vi "Crop Video Utility.vi"() -> ()   [LabVIEW 2017]
uses:
  LabVIEW/Controls/Time Crop Method.ctl
  LabVIEW/Controls/Annotation Type.ctl
  LabVIEW/Controls/Crop Video State.ctl
  LabVIEW/Controls/Frame Grabber Data.ctl
  <vilib>/userdefined/High Color/IMAQdx.ctl
  <vilib>/vision/Image Controls.llb/IMAQ Image.ctl
  <vilib>/vision/Avi.llb/IMAQ AVI2 Refnum.ctl
  LabVIEW/Controls/Rigid Body Info.ctl
  LabVIEW/Controls/Position.ctl
  LabVIEW/Controls/Orientation.ctl
  LabVIEW/Controls/Refnums.ctl
  LabVIEW/Controls/Dimensions.ctl
  LabVIEW/Controls/Room Dimensions.ctl
panel:
  in  "Continuous Playback":bool
  out "Number of Camera Frames":u32
  out "Camera Frame":u32
  in  "Clip Width":i32=1 caption="+/-" min=1
  in  "Annotation Type":T1 caption="Type"
  in  "Annotate":bool
  in  "Annotation":string
  out "Time elapsed (s)":dbl format="%_4g"
  in  "Step Size":i32=100
  in  "Skip Backward":bool
  in  "Skip Forward":bool
  in  "Invert Playback?":bool
  out "Cancel Save":bool
  in  "Time Crop\nMethod":T2
  in  "Save":bool
  in  "Help Crop":bool
  in  "Load":bool
  in  "Stop":bool
  out "Ultrasound Frame":T3(plugin-control)
  in  "Play":bool
  out "Video path":path
  out "Number of Playback Frames":i32
  in  "Playback Rate":dbl(knob)=10.173051878092375 min=1.0 max=100.0 scale=1.0..100.0
  in  "Frame Slider":cluster{i32, i32, i32}(slide)={0, 100, 0} scale=0.0..17201.0
  out "Saving":bool
  in  "Codec":u16(ring)=3 items=["Cinepak Codec by Radius", "Intel IYUV codec", "Microsoft Video 1", "FF Video Codec 1 (FFV1) (NI Vision)", "Motion JPEG (NI Vision)", "Y800 Uncompressed Grey Scale (NI Vision)", "YUV 4:2:0 Planar (NI Vision)"]
  in  "Set Crop Area":bool
  in  "Clear Crop Area":bool
  # "of"
  # "of"
  # "Min"
  # "Max"
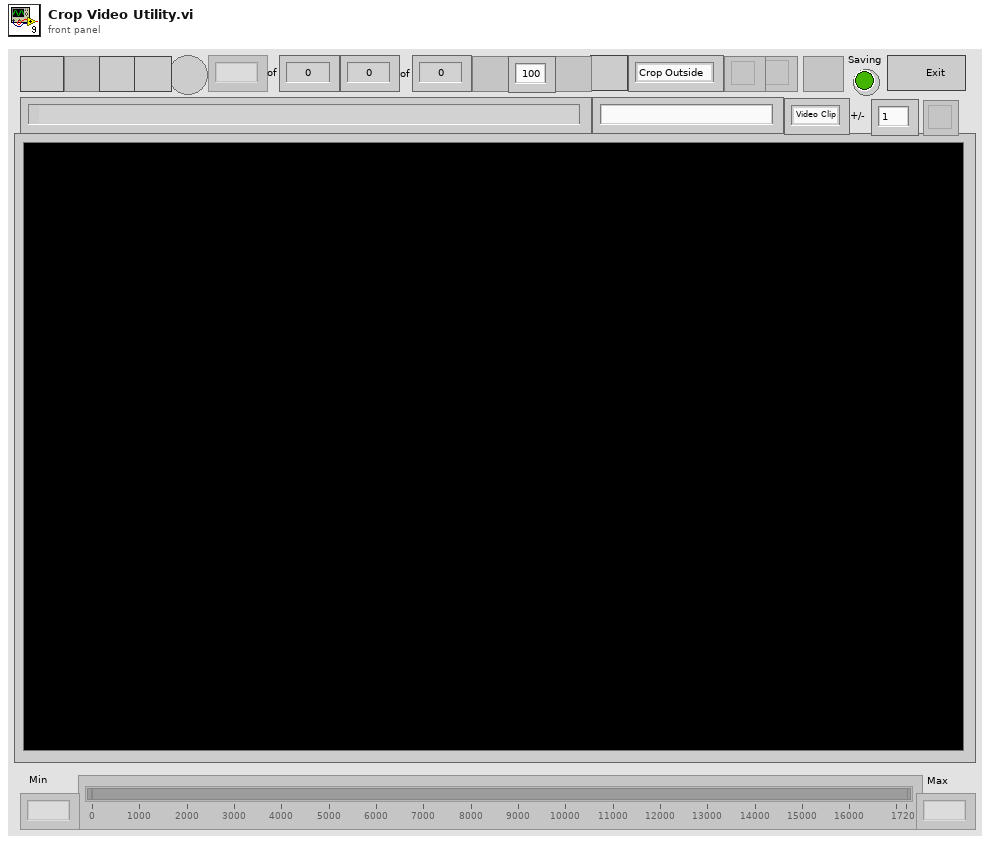
[diagram p1: front panel]
types:
  T1 = typedef "Annotation Type.ctl" = enum16{"Video Clip", "Image"}
  T2 = typedef "Time Crop Method.ctl" = enum16{"Crop Outside", "Crop Inside"}
  T3 = typedef "IMAQ Image.ctl" = refnum<image>
  T4 = typedef "Frame Grabber Data.ctl" = cluster{"Camera Session":T5, "Frame":T3, "AVI Refnum":T6, "Codecs":string[], "Frame number":u32, "Tracking File Refnum":refnum<file>, "Tick Count":u32, "Probe Object":refnum<vi>, "Playback Probe Data":dbl[][], "Rigid Body":T7, "Total no frames playback":i32, "Video FPS":dbl, "Camera connected?":bool, "Scene":refnum<vi>, "Cropped Frame":T3, "Tracker FPS":dbl, "Crop ROI":i32[], "Presentation Values":string[], "Elapsed time (ms)":u32, "Camera frames playback":u32, "Refnums":T10, "Dimensions":T11, "Playback Data As Strings":string[][], "Cropped Tracking File Refnum":refnum<file>, "Cropped AVI Refnum":T6, "Header":string[], "Total euclidian distance":dbl, "Annotation File Path":path, "Playback File Path":path, "Size per frame":dbl}
  T5 = typedef "IMAQdx.ctl" = refnum<k21>
  T6 = typedef "IMAQ AVI2 Refnum.ctl" = refnum<k20>
  T7 = typedef "Rigid Body Info.ctl" = cluster{"Position":T8, "Orientation":T9, "Quaternion":cluster{"qx":sgl, "qy":sgl, "qz":sgl, "qw":sgl}, "Tracked?":bool}
  T8 = typedef "Position.ctl" = cluster{"x (mm)":sgl, "y (mm)":sgl, "z (mm)":sgl}
  T9 = typedef "Orientation.ctl" = cluster{"Pitch (rad)":sgl, "Yaw (rad)":sgl, "Roll (rad)":sgl}
  T10 = typedef "Refnums.ctl" = cluster{"Live Refnum":refnum<vi>, "Record Refnum":refnum<vi>, "Playback Refnum":refnum<vi>, "Frame Slider Refnum":refnum<vi>, "Pause Refnum":refnum<vi>, "Home Refnum":refnum<vi>, "Crop Refnum":refnum<vi>, "Clear Crop Refnum":refnum<vi>, "stop refnum":refnum<vi>, "Playback Rate Refnum":refnum<vi>, "Presentation Refnum":refnum<vi>, "Crop Time Frame Slider Refnum":refnum<vi>, "Cancel Save Refnum":refnum<vi>, "Reverse Playback Refnum":refnum<vi>, "Recording Settings Refnum":refnum<vi>, "Camera Frame Refnum":refnum<vi>, "Continuous Playback Refnum":refnum<vi>}
  T11 = typedef "Dimensions.ctl" = cluster{"Probe Dimensions":cluster{"Probe Width":sgl, "Probe Depth":sgl, "Probe Height":sgl}, "Room Dimensions":T12}
  T12 = typedef "Room Dimensions.ctl" = cluster{"Room Width":dbl, "Room Depth":dbl, "Room Height":dbl}
  T13 = typedef "Crop Video State.ctl" = enum16{"Init", "Wait", "Load", "Playback Frame", "Save", "Close", "Set Crop Area", "Reset Crop Area", "Crop Inside", "Crop Outside", "Annotate Frame", "Annotate Clip", "Error Handling", "Shutdown"}
  T14 = typedef "Semaphore RefNum" = refnum<k1>
  T15 = enum8{"Enabled", "Disabled", "Disabled and Grayed Out"}
  T16 = typedef "Image Type" = u32
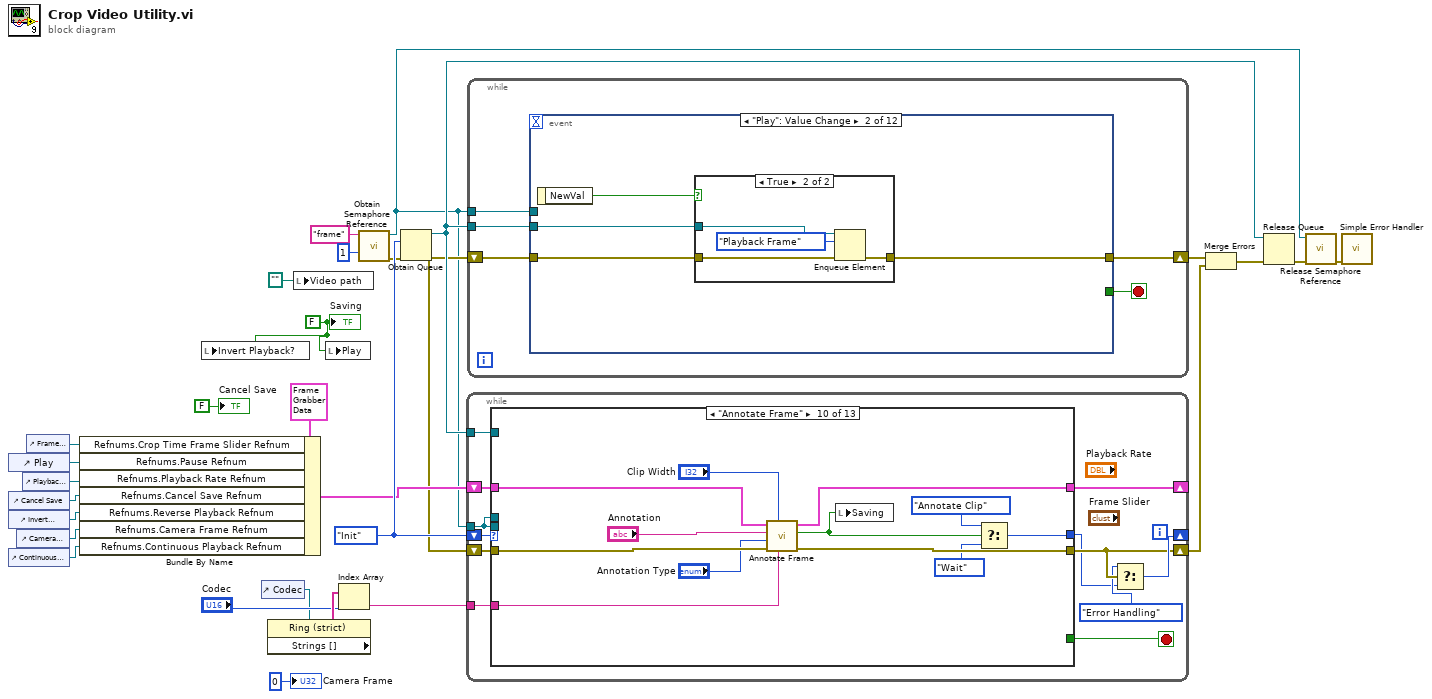
[diagram p0: block diagram]
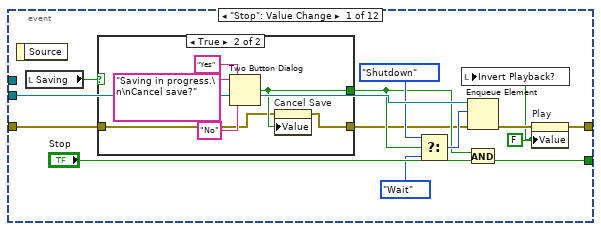
[diagram p2: hidden frame]
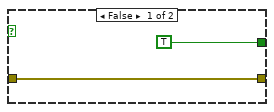
[diagram p3: hidden frame]
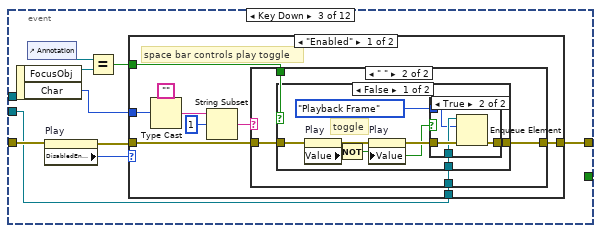
[diagram p5: hidden frame]
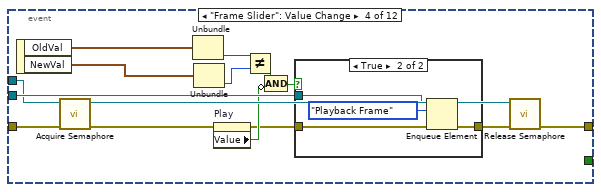
[diagram p10: hidden frame]
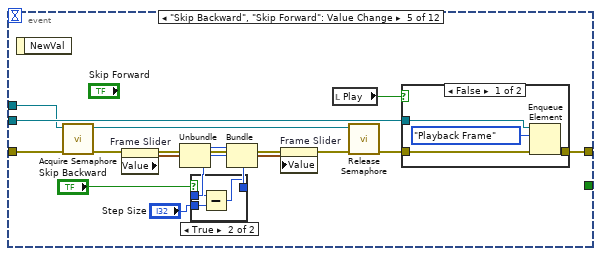
[diagram p12: hidden frame]
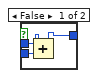
[diagram p14: hidden frame]
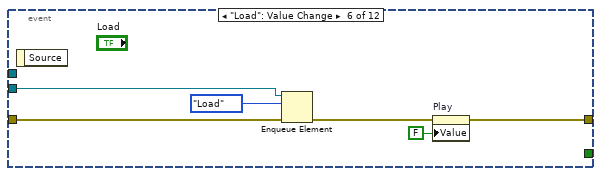
[diagram p15: hidden frame]
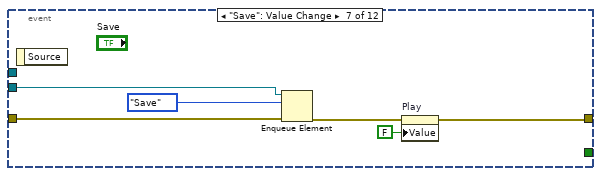
[diagram p16: hidden frame]
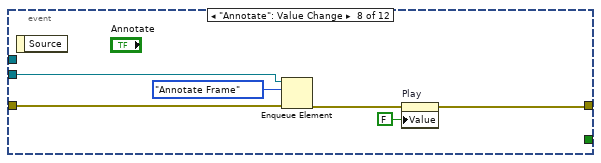
[diagram p17: hidden frame]
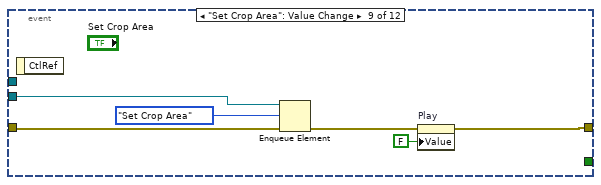
[diagram p18: hidden frame]
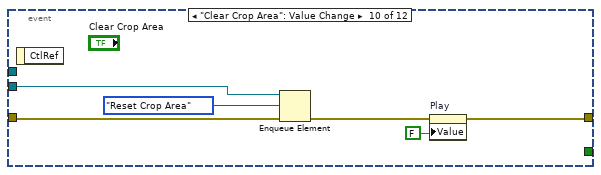
[diagram p19: hidden frame]
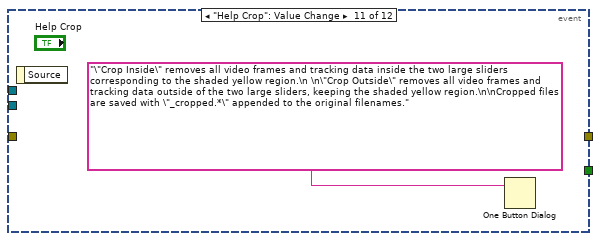
[diagram p20: hidden frame]
diagram:
  w29 = Crop_Video_State."Init" ("State")
  w11 = FALSE ("Saving")
  n1 = control-ref of="Play"() -> (w24:refnum<vi>)
  n2 = control-ref of="Cancel Save"() -> (w12:refnum<vi>)
  n3 = control-ref of="Invert Playback?"() -> (w10:refnum<vi>)
  n4 = control-ref of="Continuous Playback"() -> (w1:refnum<vi>)
  n5 = control-ref of="Camera Frame"() -> (w3:refnum<vi>)
  n6 = control-ref of="Playback Rate"() -> (w23:refnum<vi>)
  n7 = control-ref of="Frame Slider"() -> (w18:refnum<vi>)
  n8 = Bundle By Name(cluster=T4 {"Camera Session"="", "Frame"=refnum, "AVI Refnum"=refnum, "Codecs"=[], "Frame number"=0, "Tracking File Refnum"=refnum, "Tick Count"=0, "Probe Object"=refnum, "Playback Probe Data"=[], "Rigid Body"={"Position"={"x (mm)"=0.0, "y (mm)"=0.0, "z (mm)"=0.0}, "Orientation"={"Pitch (rad)"=0.0, "Yaw (rad)"=0.0, "Roll (rad)"=0.0}, "Quaternion"={"qx"=0.0, "qy"=0.0, "qz"=0.0, "qw"=0.0}, "Tracked?"=FALSE}, "Total no frames playback"=0, "Video FPS"=0.0, "Camera connected?"=FALSE, "Scene"=refnum, "Cropped Frame"=refnum, "Tracker FPS"=0.0, "Crop ROI"=[], "Presentation Values"=[], "Elapsed time (ms)"=0, "Camera frames playback"=0, "Refnums"={"Live Refnum"=refnum, "Record Refnum"=refnum, "Playback Refnum"=refnum, "Frame Slider Refnum"=refnum, "Pause Refnum"=refnum, "Home Refnum"=refnum, "Crop Refnum"=refnum, "Clear Crop Refnum"=refnum, "stop refnum"=refnum, "Playback Rate Refnum"=refnum, "Presentation Refnum"=refnum, "Crop Time Frame Slider Refnum"=refnum, "Cancel Save Refnum"=refnum, "Reverse Playback Refnum"=refnum, "Recording Settings Refnum"=refnum, "Camera Frame Refnum"=refnum, "Continuous Playback Refnum"=refnum}, "Dimensions"={"Probe Dimensions"={"Probe Width"=0.0, "Probe Depth"=1.0, "Probe Height"=0.0}, "Room Dimensions"={"Room Width"=0.0, "Room Depth"=0.0, "Room Height"=0.0}}, "Playback Data As Strings"=[], "Cropped Tracking File Refnum"=refnum, "Cropped AVI Refnum"=refnum, "Header"=[], "Total euclidian distance"=0.0, "Annotation File Path"=path "", "Playback File Path"=path "", "Size per frame"=0.0} ("Frame Grabber Data 2"), "Refnums.Crop Time Frame Slider Refnum"=w18, "Refnums.Pause Refnum"=w24, "Refnums.Playback Rate Refnum"=w23, "Refnums.Cancel Save Refnum"=w12, "Refnums.Reverse Playback Refnum"=w10, "Refnums.Camera Frame Refnum"=w3, "Refnums.Continuous Playback Refnum"=w1) -> (w21:T4)
  n9 = local write "Invert Playback?"(w11) -> ()
  n10 = control-ref of="Codec"() -> (w14:refnum<vi>)
  n11 = property class="Ring (strict)"(reference=w14) -> ("Strings []"=w17:string[])  [unwired: 1 in, 2 out]
  n12 = local write "Video path"(path "") -> ()
  n13 = local write "Play"(w11) -> ()
  n14 = Index Array(array=w17, index="Codec") -> (element=w16:string)
  n15 = call <vilib>:"Obtain Semaphore Reference.vi"("size (1)"=1, "name (unnamed)"="frame") -> ("error out"=w6:errorcluster, "semaphore"=w4:T14)  [unwired: 3 in, 1 out]
  n16 = Obtain Queue(element data type=w29, error in (no error)=w6) -> (queue out=w25:refnum<queue>, error out=w20:errorcluster)  [unwired: 3 in, 1 out]
  n17 = while {
    shift-right: [w36] -> _
    shift-left: w21 -> [w37]
    tunnel: w25 -> [w39]
    shift-right: [w34] -> w27
    shift-left: w20 -> [w38]
    shift-right: [w35] -> _
    shift-left: w29 -> [w41]
    tunnel: w16 -> [w32]
    tunnel: w4 -> [w30]
    stop <- w40 stop-if-true
    n18 = case shown="\"Annotate Frame\"" w41 {
      selector: w41 -> [_ _ _ _ _ _ _ _ _ _ w272 _ w311]
      tunnel: [_ _ _ _ _ _ _ _ _ _ _ _ w304] -> w40
      tunnel: w39 -> [_ w69 _ _ _ _ _ _ _ _ _ _ _]
      tunnel: w38 -> [w54 w68 w83 w118 w126 w135 w173 w193 w226 w255 w276 w293 w308]
      tunnel: [w55 w67 w76 w112 w121 w131 w167 w207 w233 w254 w279 w291 w310] -> w34
      tunnel: [Crop_Video_State."Wait" ("State") w66 w75 Crop_Video_State."Wait" ("State") Crop_Video_State."Wait" ("State") w140 w166 Crop_Video_State."Close" ("State") Crop_Video_State."Close" ("State") w248 Crop_Video_State."Wait" ("State") Crop_Video_State."Close" ("State") Crop_Video_State."Wait" ("State")] -> w31
      tunnel: w37 -> [w62 w65 w78 w117 w124 w138 w174 w195 w232 w252 w273 w288 w312]
      tunnel: [w59 w65 w80 w116 w125 w137 w171 w209 w235 w251 w267 w288 w303] -> w36
      tunnel: w32 -> [_ _ _ _ _ _ w172 _ _ w244 _ _ _]
      tunnel: w30 -> [_ _ _ _ _ _ _ _ _ _ _ _ _]
      tunnel: w30 -> [_ _ _ _ _ w132 _ _ _ _ _ _ _]
      frame "Init" {
        w48 = T15."Disabled and Grayed Out" ("Disabled")
        w53 = u32 100 ("Frame")
        w52 = u32 0 ("Min")
        w42 = T16 4 items=["Grayscale (U8)", "Grayscale (I16)", "Grayscale (SGL)", "Complex (CSG)", "RGB (U32)", "HSL (U32)", "RGB (U64)", "Grayscale (U16)"] ("Image Type")
        n19 = property on="Play" class="Bool (strict)"(error in=w54, "DisabledEnum"=w48) -> (error out=w51:errorcluster)  [unwired: 1 in, 1 out]
        n20 = property on="Set Crop Area" class="Bool"(error in=w51, "DisabledEnum"=w48) -> (error out=w50:errorcluster)  [unwired: 1 in, 1 out]
        n21 = property on="Clear Crop Area" class="Bool"(error in=w50, "DisabledEnum"=w48) -> (error out=w49:errorcluster)  [unwired: 1 in, 1 out]
        n22 = property on="Save" class="Bool"(error in=w49, "DisabledEnum"=w48) -> (error out=w47:errorcluster)  [unwired: 1 in, 1 out]
        n23 = property on="Frame Slider" class="Slide (strict)"(error in=w47, "DisabledEnum"=w48) -> (error out=w46:errorcluster)  [unwired: 1 in, 1 out]
        n24 = call "IMAQ Create"("Image Name"="cropped frame", "Image Type"=w42, "error in (no error)"=w46) -> ("New Image"=w43:T3, "error out"=w45:errorcluster)  [unwired: 2 in]
        n25 = Bundle(cluster=cluster{"Min":u32, "Max":u32, "Frame":u32} {"Min"=24, "Max"=167, "Frame"=33} ("Frame Slider"), "Min"=w52, "Max"=w53, "Frame"=w52) -> (w58:cluster{"Min":u32, "Max":u32, "Frame":u32})
        n26 = call "IMAQ Create"("Image Name"="frame", "Image Type"=w42, "error in (no error)"=w45) -> ("New Image"=w61:T3, "error out"=w56:errorcluster)  [unwired: 2 in]
        n27 = Bundle By Name(cluster=w62, "Cropped Frame"=w43, "Frame"=w61) -> (w59:T4)
        n28 = property on="Frame Slider" class="Slide (strict)"(error in=w56, "Value"=w58, "Scale.Minimum"=w52, "Scale.Maximum"=w53) -> (error out=w55:errorcluster)  [unwired: 1 in, 1 out]
      }
      frame "Wait", Default {
        n29 = local write "Play"(FALSE) -> ()
        n30 = Dequeue Element(queue=w69, error in (no error)=w68) -> (element=w66:T13, error out=w67:errorcluster)  [unwired: 1 in, 2 out]
      }
      frame "Load" {
        n31 = call "Open Playback Files Cropping.vi"("error in (no error)"=w83, "Frame Grabber Data In"=w78) -> ("error out"=w81:errorcluster, "Playback Video"=w82:path, "both exist and open?"=w77:bool, "Frame Grabber Data Out"=w79:T4, "Number of Playback Frames"=w74:i32, "Number of Camera Frames"=w71:u32)  [unwired: 4 in]
        n32 = Decrement(x=w71) -> (x-1=→"Number of Camera Frames":u32)
        n33 = Decrement(x=w74) -> (x-1=→"Number of Playback Frames":i32)
        n34 = case shown="True" w77 {
          tunnel: w82 -> [w87 _]
          tunnel: w81 -> [w90 w103]
          tunnel: [w96 w109] -> w80
          tunnel: w79 -> [w96 w109]
          tunnel: w78 -> [_ _]
          tunnel: [w85 w99] -> w76
          tunnel: [Crop_Video_State."Playback Frame" ("State") Crop_Video_State."Wait" ("State")] -> w75
          tunnel: [w87 _] -> w73
          frame True {
            w84 = T15."Enabled" ("Disabled")
            n35 = property on="Skip Backward" class="Bool"(error in=w90, "DisabledEnum"=w84) -> (error out=w89:errorcluster)  [unwired: 1 in, 1 out]
            n36 = property on="Skip Forward" class="Bool"(error in=w89, "DisabledEnum"=w84) -> (error out=w88:errorcluster)  [unwired: 1 in, 1 out]
            n37 = property on="Play" class="Bool (strict)"(error in=w88, "DisabledEnum"=w84) -> (error out=w93:errorcluster)  [unwired: 1 in, 1 out]
            n38 = property on="Set Crop Area" class="Bool"(error in=w93, "DisabledEnum"=w84) -> (error out=w92:errorcluster)  [unwired: 1 in, 1 out]
            n39 = property on="Save" class="Bool"(error in=w92, "DisabledEnum"=w84) -> (error out=w91:errorcluster)  [unwired: 1 in, 1 out]
            n40 = local write "Play"(TRUE ("Play")) -> ()
            n41 = property on="Frame Slider" class="Slide (strict)"(error in=w91, "DisabledEnum"=w84) -> (error out=w86:errorcluster)  [unwired: 1 in, 1 out]
            n42 = property on="Annotate" class="Bool"(error in=w86, "DisabledEnum"=w84) -> (error out=w85:errorcluster)  [unwired: 1 in, 1 out]
          }
          frame False {
            w97 = T15."Disabled and Grayed Out" ("Disabled")
            n43 = property on="Skip Backward" class="Bool"(error in=w103, "DisabledEnum"=w97) -> (error out=w102:errorcluster)  [unwired: 1 in, 1 out]
            n44 = property on="Skip Forward" class="Bool"(error in=w102, "DisabledEnum"=w97) -> (error out=w101:errorcluster)  [unwired: 1 in, 1 out]
            n45 = property on="Play" class="Bool (strict)"(error in=w101, "DisabledEnum"=w97) -> (error out=w106:errorcluster)  [unwired: 1 in, 1 out]
            n46 = property on="Set Crop Area" class="Bool"(error in=w106, "DisabledEnum"=w97) -> (error out=w105:errorcluster)  [unwired: 1 in, 1 out]
            n47 = property on="Save" class="Bool"(error in=w105, "DisabledEnum"=w97) -> (error out=w104:errorcluster)  [unwired: 1 in, 1 out]
            n48 = One Button Dialog(message="Could not open files for playback.") -> ()  [unwired: 1 in, 1 out]
            n49 = local write "Play"(TRUE ("Play")) -> ()
            n50 = property on="Frame Slider" class="Slide (strict)"(error in=w104, "DisabledEnum"=w97) -> (error out=w98:errorcluster)  [unwired: 1 in, 1 out]
            n51 = property on="Annotate" class="Bool"(error in=w98, "DisabledEnum"=w97) -> (error out=w99:errorcluster)  [unwired: 1 in, 1 out]
          }
        }
        "Video path" <- w73
      }
      frame "Set Crop Area" {
        n52 = call "Set Crop ROI.vi"("error in (no error)"=w118, "Frame Grabber Data in"=w117) -> ("error out"=w110:errorcluster, "Image Out"=w115:T3, "Frame Grabber Data out"=w116:T4, "Zero crop size?"=w111:bool)  [unwired: 5 in, 1 out]
        n53 = local write "Ultrasound Frame"(w115) -> ()
        n54 = case shown="True" w111 {
          frame False {
          }
          frame True {
            n55 = One Button Dialog(message="Warning: invalid crop area.") -> ()  [unwired: 1 in, 1 out]
          }
        }
        n56 = property on="Clear Crop Area" class="Bool"(error in=w110, "DisabledEnum"=T15."Enabled" ("Disabled")) -> (error out=w112:errorcluster)  [unwired: 1 in, 1 out]
      }
      frame "Reset Crop Area" {
        n57 = call "Clear Crop ROI.vi"("error in (no error)"=w126, "Frame Grabber Data in"=w124) -> ("error out"=w121:errorcluster, "Image Out"=w123:T3, "Frame Grabber Data out"=w125:T4)  [unwired: 6 in, 1 out]
        n58 = local write "Ultrasound Frame"(w123) -> ()
        n59 = property on="Clear Crop Area" class="Bool"(error in=w121, "DisabledEnum"=T15."Disabled and Grayed Out" ("Disabled")) -> ()  [unwired: 1 in, 2 out]
      }
      frame "Playback Frame" {
        n60 = call "Playback Frame Cropping.vi"("error in (no error)"=w135, "Frame Grabber Data in"=w138) -> ("error out"=w133:errorcluster, "Continue playback?"=w130:bool, "Image"=→"Ultrasound Frame":T3, "Frame Grabber Data out"=w137:T4, "Time elapsed (s)"=→"Time elapsed (s)":dbl)  [unwired: 4 in, 1 out]
        n61 = case shown="True" w130 {
          selector: w130 -> [w143 w145]
          tunnel: [w144 w147] -> w131
          tunnel: "Invert Playback?" -> [_ w152]
          tunnel: w133 -> [w144 w151]
          tunnel: w132 -> [_ w150]
          tunnel: [w143 w145] -> w129
          frame False {
          }
          frame True {
            n62 = call <vilib>:"Acquire Semaphore.vi"("error in (no error)"=w151, "semaphore"=w150) -> ("error out"=w149:errorcluster, "semaphore out"=w146:T14)  [unwired: 3 in, 1 out]
            n63 = property on="Frame Slider" class="Slide (strict)"(error in=w149) -> (error out=w155:errorcluster, "Value"=w158:cluster{i32, i32, i32})  [unwired: 1 in, 1 out]
            n64 = Unbundle(w158) -> (w157:i32, w156:i32, w154:i32)
            n65 = case shown="True" w152 {
              tunnel: w154 -> [w161 w162]
              tunnel: [w160 w163] -> w153
              frame False {
                n66 = Increment(x=w161) -> (x+1=w160:i32)
              }
              frame True {
                n67 = Decrement(x=w162) -> (x-1=w163:i32)
              }
            }
            n68 = Bundle(w157, w156, w153) -> (w159:cluster{i32, i32, i32})  [unwired: 1 in]
            n69 = property on="Frame Slider" class="Slide (strict)"(error in=w155, "Value"=w159) -> (error out=w148:errorcluster)  [unwired: 1 in, 1 out]
            n70 = call <vilib>:"Release Semaphore.vi"("error in (no error)"=w148, "semaphore"=w146) -> ("error out"=w147:errorcluster)  [unwired: 4 in, 1 out]
          }
        }
        n71 = And(x="Play", y=w129) -> (x .and. y?=w128:bool)
        n72 = Select(t=Crop_Video_State."Playback Frame" ("State"), s=w128, f=Crop_Video_State."Wait" ("State")) -> (s? t:f=w140:T13)
      }
      frame "Save" {
        n73 = call "Configure Crop.vi"("Codec"=w172, "error in (no error)"=w173, "Time Crop Method"="Time Crop\nMethod", "Frame Grabber Data In"=w174) -> ("error out"=w169:errorcluster, "Valid crop region?"=w170:bool, "Saving?"=w164:bool, "Frame Grabber Data Out"=w171:T4)  [unwired: 4 in]
        n74 = local write "Saving"(w164) -> ()
        n75 = And(x=w164, y=w170) -> (x .and. y?=w165:bool)
        n76 = case shown="True" w165 {
          tunnel: w169 -> [w175 w187]
          tunnel: "Time Crop\nMethod" -> [_ w189]
          tunnel: [Crop_Video_State."Wait" ("State") w188] -> w166
          tunnel: [w175 w179] -> w167
          frame False {
            n77 = One Button Dialog(message="Invalid time crop region/save cancelled by user.") -> ()  [unwired: 1 in, 1 out]
          }
          frame True {
            w178 = T15."Disabled and Grayed Out" ("Disabled")
            n78 = property on="Set Crop Area" class="Bool"(error in=w187, "DisabledEnum"=w178) -> (error out=w186:errorcluster)  [unwired: 1 in, 1 out]
            n79 = property on="Save" class="Bool"(error in=w186, "DisabledEnum"=w178) -> (error out=w185:errorcluster)  [unwired: 1 in, 1 out]
            n80 = property on="Load" class="Bool"(error in=w185, "DisabledEnum"=w178) -> (error out=w184:errorcluster)  [unwired: 1 in, 1 out]
            n81 = property on="Frame Slider" class="Slide (strict)"(error in=w184, "DisabledEnum"=w178) -> (error out=w183:errorcluster)  [unwired: 1 in, 1 out]
            n82 = property on="Clear Crop Area" class="Bool"(error in=w183, "DisabledEnum"=w178) -> (error out=w181:errorcluster)  [unwired: 1 in, 1 out]
            n83 = property on="Load" class="Bool"(error in=w181, "DisabledEnum"=w178) -> (error out=w182:errorcluster)  [unwired: 1 in, 1 out]
            n84 = case shown="\"Crop Outside\", Default" w189 {
              tunnel: [Crop_Video_State."Crop Inside" ("t") Crop_Video_State."Crop Outside" ("t")] -> w188
              frame "Crop Inside" {
              }
              frame "Crop Outside", Default {
              }
            }
            n85 = property on="Play" class="Bool (strict)"(error in=w182, "DisabledEnum"=w178) -> (error out=w180:errorcluster)  [unwired: 1 in, 1 out]
            n86 = property on="Annotate" class="Bool"(error in=w180, "DisabledEnum"=w178) -> (error out=w179:errorcluster)  [unwired: 1 in, 1 out]
          }
        }
      }
      frame "Crop Inside" {
        w202 = u32 0 ("Starting frame number")
        n87 = property on="Frame Slider" class="Slide (strict)"(error in=w193) -> (error out=w192:errorcluster, "Value"=w194:cluster{i32, i32, i32})  [unwired: 1 in, 1 out]
        n88 = Bundle By Name(cluster=w195, "Frame number"=w202) -> (w196:T4)
        n89 = Unbundle By Name(w195) -> ("Total no frames playback"=w205:i32)
        n90 = Unbundle(w194) -> (w198:i32, w199:i32)  [unwired: 1 out]
        n91 = for {
          N: w198 -> [_]
          shift-right: [w220] -> w204
          shift-left: w192 -> [w221]
          shift-right: [w218] -> w201
          shift-left: w196 -> [w219]
          tunnel: w202 -> [w217]
          stop <- w216 stop-if-true
          # "First portion"
          n92 = call "Record Frame Crop.vi"("error in (no error)"=w221, "Starting frame number"=w217, "Frame Grabber Data In in"=w219) -> ("error out"=w220:errorcluster, "Cancel save?"=w216:bool, "Frame Grabber Data out"=w218:T4)  [unwired: 6 in]
        }
        n93 = Bundle By Name(cluster=w201, "Frame number"=w199) -> (w200:T4)
        n94 = Subtract(x=w199, y=w198) -> (x-y=w197:i32)
        n95 = Subtract(x=w205, y=w199) -> (x-y=w203:i32)
        n96 = for {
          N: w203 -> [_]
          shift-right: [w214] -> w208
          shift-left: w204 -> [w215]
          shift-right: [w212] -> w209
          shift-left: w200 -> [w213]
          tunnel: w197 -> [w211]
          stop <- w210 stop-if-true
          # "Second portion"
          n97 = call "Record Frame Crop.vi"("error in (no error)"=w215, "Starting frame number"=w211, "Frame Grabber Data In in"=w213) -> ("error out"=w214:errorcluster, "Cancel save?"=w210:bool, "Frame Grabber Data out"=w212:T4)  [unwired: 6 in]
        }
        n98 = flat-sequence {
          tunnel: w208 -> [w222]
          tunnel: [w222] -> w207
          frame #0 {
            n99 = local write "Saving"(FALSE) -> ()
          }
        }
      }
      frame "Crop Outside" {
        n100 = property on="Frame Slider" class="Slide (strict)"(error in=w226) -> (error out=w224:errorcluster, "Value"=w225:cluster{i32, i32, i32})  [unwired: 1 in, 1 out]
        n101 = Unbundle(w225) -> (w227:i32, w230:i32)  [unwired: 1 out]
        n102 = Bundle By Name(cluster=w232, "Frame number"=w227) -> (w228:T4)
        n103 = Subtract(x=w230, y=w227) -> (x-y=w229:i32)
        n104 = for {
          N: w229 -> [_]
          shift-right: [w240] -> w234
          shift-left: w224 -> [w241]
          tunnel: w227 -> [w239]
          shift-right: [w238] -> w235
          shift-left: w228 -> [w237]
          stop <- w236 stop-if-true
          # "Middle portion"
          n105 = call "Record Frame Crop.vi"("error in (no error)"=w241, "Starting frame number"=w239, "Frame Grabber Data In in"=w237) -> ("error out"=w240:errorcluster, "Cancel save?"=w236:bool, "Frame Grabber Data out"=w238:T4)  [unwired: 6 in]
        }
        n106 = flat-sequence {
          tunnel: w234 -> [w243]
          tunnel: [w243] -> w233
          frame #0 {
            n107 = local write "Saving"(FALSE) -> ()
          }
        }
      }
      frame "Annotate Frame" {
        n108 = call "Annotate Frame.vi"("Codec"=w244, "Clip width"="Clip Width", "error in (no error)"=w255, "Annotation Type"="Annotation Type", "Annotation"="Annotation", "Frame Grabber Data In in"=w252) -> ("error out"=w254:errorcluster, "saving?"=w250:bool, "Frame Grabber Data Out"=w251:T4)  [unwired: 3 in]
        n109 = local write "Saving"(w250) -> ()
        n110 = Select(t=Crop_Video_State."Annotate Clip" ("State"), s=w250, f=Crop_Video_State."Wait" ("State")) -> (s? t:f=w248:T13)
      }
      frame "Annotate Clip" {
        # "reset"
        n111 = local read "Clip Width"() -> (w266:i32)
        n112 = Unbundle By Name(w273) -> ("Tracker FPS"=w263:dbl, "Video FPS"=w262:dbl, "Frame number"=w259:u32)
        n113 = Multiply(x=w266, y=2) -> (x*y=w274:i32)
        n114 = To Double Precision Float(number=w259) -> (double precision float=w260:dbl)
        n115 = Divide(x=w263, y=w262) -> (x/y=w257:dbl)
        n116 = Quotient & Remainder(x=w260, y=w257) -> (floor(x/y)=w258:dbl)  [unwired: 1 out]
        n117 = Multiply(x=w257, y=w258) -> (x*y=w256:dbl)
        n118 = Multiply(x=w274, y=w257) -> (x*y=w264:dbl)
        n119 = Multiply(x=w266, y=w257) -> (x*y=w261:dbl)
        n120 = Subtract(x=w256, y=w261) -> (x-y=w265:dbl)
        n121 = Bundle By Name(cluster=w273, "Frame number"=w265) -> (w277:T4)
        n122 = for {
          N: w264 -> [_]
          shift-right: [w284] -> w271
          shift-left: w276 -> [w285]
          shift-right: [w283] -> w269
          shift-left: w277 -> [w282]
          stop <- w281 stop-if-true
          # "Middle portion"
          n123 = call "Record Frame Crop.vi"("error in (no error)"=w285, "Starting frame number"=u32 0, "Frame Grabber Data In in"=w282) -> ("error out"=w284:errorcluster, "Cancel save?"=w281:bool, "Frame Grabber Data out"=w283:T4)  [unwired: 6 in]
        }
        n124 = call "Close Files.vi"("error in (no error)"=w271, "State"=w272, "Frame Grabber Data in"=w269) -> ("error out"=w270:errorcluster, "Frame Grabber Data Out"=w268:T4)  [unwired: 5 in, 2 out]
        n125 = Bundle By Name(cluster=w268, "Frame number"=w259) -> (w267:T4)
        n126 = flat-sequence {
          tunnel: [w286] -> _
          tunnel: [w286] -> w279
          tunnel: w270 -> [w286]
          frame #0 {
            n127 = local write "Saving"(FALSE) -> ()
          }
        }
      }
      frame "Error Handling" {
        n128 = call <vilib>:"Simple Error Handler.vi"("error in (no error)"=w293) -> ("error out"=w292:errorcluster)  [unwired: 4 in, 4 out]
        n129 = local write "Play"(FALSE ("Play")) -> ()
        n130 = call <vilib>:"Clear Errors.vi"("error in (no error)"=w292) -> ("error out"=w291:errorcluster)  [unwired: 5 in, 1 out]
      }
      frame "Close", "Shutdown" {
        w295 = T15."Disabled and Grayed Out" ("Disabled")
        n131 = call "Close Files.vi"("error in (no error)"=w308, "State"=w311, "Frame Grabber Data in"=w312) -> ("error out"=w300:errorcluster, "Shutdown?"=w304:bool, "File Path Control"=w302:path, "Frame Grabber Data Out"=w303:T4)  [unwired: 5 in]
        n132 = property on="Skip Backward" class="Bool"(error in=w300, "DisabledEnum"=w295) -> (error out=w299:errorcluster)  [unwired: 1 in, 1 out]
        n133 = local write "Video path"(w302) -> ()
        n134 = local write "Camera Frame"(u32 0 ("Camera Frame")) -> ()
        n135 = property on="Skip Forward" class="Bool"(error in=w299, "DisabledEnum"=w295) -> (error out=w298:errorcluster)  [unwired: 1 in, 1 out]
        n136 = property on="Save" class="Bool"(error in=w298, "DisabledEnum"=w295) -> (error out=w307:errorcluster)  [unwired: 1 in, 1 out]
        n137 = property on="Clear Crop Area" class="Bool"(error in=w307, "DisabledEnum"=w295) -> (error out=w306:errorcluster)  [unwired: 1 in, 1 out]
        n138 = property on="Set Crop Area" class="Bool"(error in=w306, "DisabledEnum"=w295) -> (error out=w305:errorcluster)  [unwired: 1 in, 1 out]
        n139 = property on="Frame Slider" class="Slide (strict)"(error in=w305, "DisabledEnum"=w295) -> (error out=w301:errorcluster)  [unwired: 1 in, 1 out]
        n140 = property on="Play" class="Bool (strict)"(error in=w301, "DisabledEnum"=w295) -> (error out=w297:errorcluster)  [unwired: 1 in, 1 out]
        n141 = property on="Annotate" class="Bool"(error in=w297, "DisabledEnum"=w295) -> (error out=w296:errorcluster)  [unwired: 1 in, 1 out]
        n142 = property on="Load" class="Bool"(error in=w296, "DisabledEnum"=T15."Enabled" ("Disabled")) -> (error out=w310:errorcluster)  [unwired: 1 in, 1 out]
      }
    }
    n143 = Select(t=Crop_Video_State."Error Handling", s=w34, f=w31) -> (s? t:f=w35:T13)
  }
  n144 = while {
    tunnel: w25 -> [w317]
    shift-right: [w315] -> w28
    shift-left: w20 -> [w316]
    tunnel: w4 -> [w314]
    stop <- w318 stop-if-true
    n145 = event shown="[1] \"Play\": Value Change" {
      selector: _ -> [_ _ _ _ _ _ _ _ _ _ _ _]
      dyn-events: _ -> [_ _ _ _ _ _ _ _ _ _ _ _]
      timeout: _ -> [_ _ _ _ _ _ _ _ _ _ _ _]
      tunnel: [w323 _ _ _ _ _ _ _ _ _ _ _] -> w318
      tunnel: w317 -> [w330 w341 w352 w399 w424 w440 w446 w452 w459 w465 _ _]
      tunnel: w316 -> [w321 w343 w355 w398 w422 w441 w447 w453 w457 w463 _ w476]
      tunnel: [w329 w342 w356 w394 w411 w436 w443 w450 w454 w460 _ w475] -> w315
      tunnel: w314 -> [_ _ _ w397 w423 _ _ _ _ _ _ _]
      event "Stop": Value Change {
        w319 = FALSE ("Play")
        n146 = event-data() -> ()  [unwired: 1 in, 1 out]
        n147 = local read "Saving"() -> (w327:bool)
        n148 = case shown="True" w327 {
          tunnel: [TRUE ("T button?") w336] -> w322
          tunnel: w321 -> [w332 w335]
          tunnel: [w332 w334] -> w320
          frame False {
          }
          frame True {
            n149 = Two Button Dialog(message="Saving in progress.\n\nCancel save?", 1:"No" ("F button name (\"Cancel\")"), 2:"Yes" ("T button name (\"OK\")")) -> (T button?=w336:bool)
            n150 = property on="Cancel Save" class="Bool (strict)"(error in=w335, "Value"=w336) -> (error out=w334:errorcluster)  [unwired: 1 in, 1 out]
          }
        }
        n151 = Select(t=Crop_Video_State."Shutdown" ("element"), s=w322, f=Crop_Video_State."Wait") -> (s? t:f=w325:T13)
        n152 = local write "Invert Playback?"(w319) -> ()
        n153 = Enqueue Element(queue=w330, element=w325, error in (no error)=w320) -> (error out=w328:errorcluster)  [unwired: 1 in, 2 out]
        n154 = And(x=w322, y="Stop") -> (x .and. y?=w323:bool)
        n155 = property on="Play" class="Bool (strict)"(error in=w328, "Value"=w319) -> (error out=w329:errorcluster)  [unwired: 1 in, 1 out]
      }
      event "Play": Value Change {
        n156 = event-data() -> ("NewVal"=w340:bool)  [unwired: 1 in]
        n157 = case shown="True" w340 {
          tunnel: w343 -> [w344 w348]
          tunnel: [w344 w347] -> w342
          tunnel: w341 -> [_ w346]
          frame False {
          }
          frame True {
            n158 = Enqueue Element(queue=w346, element=Crop_Video_State."Playback Frame", error in (no error)=w348) -> (error out=w347:errorcluster)  [unwired: 1 in, 2 out]
          }
        }
      }
      event Key Down {
        n159 = event-data() -> ("FocusObj"=w351:refnum<vi>, "Char"=w357:i16)  [unwired: 1 in]
        n160 = control-ref of="Annotation"() -> (w350:refnum<vi>)
        n161 = property on="Play" class="Bool (strict)"(error in=w355) -> (error out=w354:errorcluster, "DisabledEnum"=w353:T15)  [unwired: 1 in, 1 out]
        n162 = Equal?(x=w350, y=w351) -> (x = y?=w349:bool)
        n163 = case shown="\"Enabled\"" w353 {
          tunnel: w357 -> [w364 _]
          tunnel: w354 -> [w361 w386]
          tunnel: [w360 w386] -> w356
          tunnel: w352 -> [w359 _]
          tunnel: w349 -> [w358 _]
          frame "Enabled" {
            # "space bar controls play toggle"
            n164 = Type Cast(type="", x=w364) -> (*(type *) &x=w366:string)
            n165 = String Subset(string=w366, offset (0)=1) -> (substring=w362:string)  [unwired: 1 in]
            n166 = case shown="\" \"" w362 {
              tunnel: w361 -> [w367 w371]
              tunnel: [w367 w370] -> w360
              tunnel: w359 -> [_ w369]
              tunnel: w358 -> [_ w368]
              frame Default {
                # "do nothing"
              }
              frame " " {
                n167 = case shown="False" w368 {
                  tunnel: w371 -> [w379 w385]
                  tunnel: [w375 w385] -> w370
                  tunnel: w369 -> [w374 _]
                  frame False {
                    # "toggle"
                    n168 = property on="Play" class="Bool (strict)"(error in=w379) -> (error out=w377:errorcluster, "Value"=w378:bool)  [unwired: 1 in, 1 out]
                    n169 = Not(x=w378) -> (.not. x?=w373:bool)
                    n170 = property on="Play" class="Bool (strict)"(error in=w377, "Value"=w373) -> (error out=w376:errorcluster)  [unwired: 1 in, 1 out]
                    n171 = case shown="True" w373 {
                      tunnel: w376 -> [w380 w384]
                      tunnel: [w380 w383] -> w375
                      tunnel: w374 -> [_ w382]
                      tunnel: Crop_Video_State."Playback Frame" ("State") -> [_ w381]
                      frame False {
                      }
                      frame True {
                        n172 = Enqueue Element(queue=w382, element=w381, error in (no error)=w384) -> (error out=w383:errorcluster)  [unwired: 1 in, 2 out]
                      }
                    }
                  }
                  frame True {
                  }
                }
              }
            }
          }
          frame Default {
          }
        }
      }
      event "Frame Slider": Value Change {
        n173 = event-data() -> ("OldVal"=w401:cluster{i32, i32, i32}, "NewVal"=w400:cluster{i32, i32, i32})  [unwired: 1 in]
        n174 = call <vilib>:"Acquire Semaphore.vi"("error in (no error)"=w398, "semaphore"=w397) -> ("error out"=w396:errorcluster, "semaphore out"=w393:T14)  [unwired: 3 in, 1 out]
        n175 = Unbundle(w401) -> (w391:i32)  [unwired: 2 out]
        n176 = Unbundle(w400) -> (w392:i32)  [unwired: 2 out]
        n177 = property on="Play" class="Bool (strict)"(error in=w396) -> (error out=w387:errorcluster, "Value"=w388:bool)  [unwired: 1 in, 1 out]
        n178 = Not Equal?(x=w391, y=w392) -> (x != y?=w390:bool)
        n179 = Compound Arithmetic op=AND(w390, invert w388) -> (w389:bool)
        n180 = case shown="True" w389 {
          tunnel: w399 -> [_ w406]
          tunnel: w387 -> [w402 w405]
          tunnel: [w402 w404] -> w395
          frame False {
          }
          frame True {
            n181 = Enqueue Element(queue=w406, element=Crop_Video_State."Playback Frame", error in (no error)=w405) -> (error out=w404:errorcluster)  [unwired: 1 in, 2 out]
          }
        }
        n182 = call <vilib>:"Release Semaphore.vi"("error in (no error)"=w395, "semaphore"=w393) -> ("error out"=w394:errorcluster)  [unwired: 4 in, 1 out]
      }
      event "Skip Backward", "Skip Forward": Value Change {
        n183 = event-data() -> ()  [unwired: 1 in, 1 out]
        n184 = call <vilib>:"Acquire Semaphore.vi"("error in (no error)"=w422, "semaphore"=w423) -> ("error out"=w421:errorcluster, "semaphore out"=w408:T14)  [unwired: 3 in, 1 out]
        n185 = property on="Frame Slider" class="Slide (strict)"(error in=w421) -> (error out=w412:errorcluster, "Value"=w419:cluster{i32, i32, i32})  [unwired: 1 in, 1 out]
        n186 = Unbundle(w419) -> (w418:i32, w417:i32, w415:i32)
        n187 = case shown="True" "Skip Backward" {
          tunnel: "Step Size" -> [w432 w435]
          tunnel: w415 -> [w430 w434]
          tunnel: [w431 w433] -> w414
          frame False {
            n188 = Add(x=w430, y=w432) -> (x+y=w431:i32)
          }
          frame True {
            n189 = Subtract(x=w434, y=w435) -> (x-y=w433:i32)
          }
        }
        n190 = Bundle(w418, w417, w414) -> (w413:cluster{i32, i32, i32})  [unwired: 1 in]
        n191 = property on="Frame Slider" class="Slide (strict)"(error in=w412, "Value"=w413) -> (error out=w410:errorcluster)  [unwired: 1 in, 1 out]
        n192 = local read "Play"() -> (w407:bool)
        n193 = call <vilib>:"Release Semaphore.vi"("error in (no error)"=w410, "semaphore"=w408) -> ("error out"=w409:errorcluster)  [unwired: 4 in, 1 out]
        n194 = case shown="False" w407 {
          tunnel: w424 -> [w428 _]
          tunnel: [w426 w429] -> w411
          tunnel: w409 -> [w425 w429]
          frame False {
            n195 = Enqueue Element(queue=w428, element=Crop_Video_State."Playback Frame", error in (no error)=w425) -> (error out=w426:errorcluster)  [unwired: 1 in, 2 out]
          }
          frame True {
          }
        }
      }
      event "Load": Value Change {
        n196 = event-data() -> ()  [unwired: 1 in, 1 out]
        n197 = Enqueue Element(queue=w440, element=Crop_Video_State."Load", error in (no error)=w441) -> (error out=w437:errorcluster)  [unwired: 1 in, 2 out]
        n198 = property on="Play" class="Bool (strict)"(error in=w437, "Value"=FALSE ("Play")) -> (error out=w436:errorcluster)  [unwired: 1 in, 1 out]
      }
      event "Save": Value Change {
        n199 = event-data() -> ()  [unwired: 1 in, 1 out]
        n200 = Enqueue Element(queue=w446, element=Crop_Video_State."Save", error in (no error)=w447) -> (error out=w442:errorcluster)  [unwired: 1 in, 2 out]
        n201 = property on="Play" class="Bool (strict)"(error in=w442, "Value"=FALSE ("Play")) -> (error out=w443:errorcluster)  [unwired: 1 in, 1 out]
      }
      event "Annotate": Value Change {
        n202 = event-data() -> ()  [unwired: 1 in, 1 out]
        n203 = Enqueue Element(queue=w452, element=Crop_Video_State."Annotate Frame", error in (no error)=w453) -> (error out=w449:errorcluster)  [unwired: 1 in, 2 out]
        n204 = property on="Play" class="Bool (strict)"(error in=w449, "Value"=FALSE ("Play")) -> (error out=w450:errorcluster)  [unwired: 1 in, 1 out]
      }
      event "Set Crop Area": Value Change {
        n205 = event-data() -> ()  [unwired: 1 in, 1 out]
        n206 = Enqueue Element(queue=w459, element=Crop_Video_State."Set Crop Area", error in (no error)=w457) -> (error out=w456:errorcluster)  [unwired: 1 in, 2 out]
        n207 = property on="Play" class="Bool (strict)"(error in=w456, "Value"=FALSE ("Play")) -> (error out=w454:errorcluster)  [unwired: 1 in, 1 out]
      }
      event "Clear Crop Area": Value Change {
        n208 = event-data() -> ()  [unwired: 1 in, 1 out]
        n209 = Enqueue Element(queue=w465, element=Crop_Video_State."Reset Crop Area", error in (no error)=w463) -> (error out=w461:errorcluster)  [unwired: 1 in, 2 out]
        n210 = property on="Play" class="Bool (strict)"(error in=w461, "Value"=FALSE ("Play")) -> (error out=w460:errorcluster)  [unwired: 1 in, 1 out]
      }
      event "Help Crop": Value Change {
        n211 = event-data() -> ()  [unwired: 1 in, 1 out]
        n212 = One Button Dialog(message="\"Crop Inside\" removes all video frames and tracking data inside the two large sliders corresponding to the shaded yellow region.\n \n\"Crop Outside\" removes all video frames and tracking data outside of the two large sliders, keeping the shaded yellow region.\n\nCropped files are saved with \"_cropped.*\" appended to the original filenames.") -> ()  [unwired: 1 in, 1 out]
      }
      event "Annotation": Value Change {
        w469 = TRUE ("replace all? (F)")
        w468 = "_"
        # "remove spaces and periods"
        n213 = event-data() -> ("CtlRef"=w474:refnum<vi>)  [unwired: 1 in]
        n214 = property class="Str"(reference=w474, error in=w476) -> (reference out=w477:refnum<vi>, error out=w480:errorcluster, "Value"=w478:string)
        n215 = call <vilib>:"Space Constant.vi"() -> ("String"=w479:string)
        n216 = Search and Replace String(replace all?=w469, input string=w478, search string=w479, replace string=w468, error in=w480) -> (result string=w473:string, error out=w471:errorcluster)  [unwired: 3 in, 2 out]
        n217 = Search and Replace String(replace all?=w469, input string=w473, search string=".", replace string=w468, error in=w471) -> (result string=w472:string, error out=w470:errorcluster)  [unwired: 3 in, 2 out]
        n218 = property class="Str"(reference=w477, error in=w470, "Value"=w472) -> (error out=w475:errorcluster)  [unwired: 1 out]
      }
    }
  }
  n219 = Merge Errors(w28, w27) -> (w26:errorcluster)
  n220 = Release Queue(queue=w25, error in (no error)=w26) -> (error out=w8:errorcluster)  [unwired: 1 in, 2 out]
  n221 = call <vilib>:"Release Semaphore Reference.vi"("error in (no error)"=w8, "semaphore"=w4) -> ("error out"=w7:errorcluster)  [unwired: 8 in, 1 out]
  n222 = call <vilib>:"Simple Error Handler.vi"("error in (no error)"=w7) -> ()  [unwired: 4 in, 5 out]
  "Saving" <- w11
  "Cancel Save" <- FALSE ("Saving 2")
  "Camera Frame" <- u32 0 ("Camera Frame")
